vi "Auto Cleanup on Idle.vi"() -> (0 "auto cleanup":bool)   [LabVIEW 2021, in "NI Discovery V1 Client.lvlib"]
uses:
  NI Discovery V1 Client.lvlib
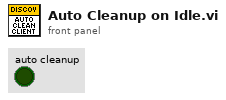
[diagram p1: front panel]
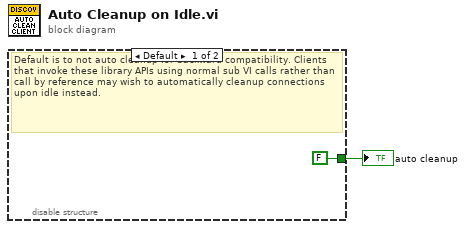
[diagram p0: block diagram]
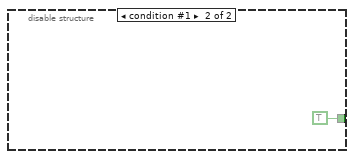
[diagram p2: hidden frame]
diagram:
  n1 = disable-structure shown="Default" {
    disable-tunnel: [FALSE TRUE] -> w1
    frame condition #0 (active) {
      # "Default is to not auto cleanup for backward compatibility. Clients that invoke these library APIs using normal sub VI calls rather than call by reference may wish to automatically cleanup connections upon idle instead."
    }
    frame condition #1 {
    }
  }
  "auto cleanup" <- w1
